vi "SaveConfigFile.vi"(0 "IP":string caption="Robot IP Address", 1 "RoboguideRobotPath":path, 2 "ConnectRoboguide":bool, 3 "Use Telnet":bool, 4 "Telnet password":string, 5 "Use FTP":bool, 6 "FTP user":string, 7 "FTP password":string, 8 "Use SNPX":bool, 9 "error in (no error)":errorcluster, 10 "Licensee":string, 12 "Key":string) -> ()   [LabVIEW 2019]
uses:
  <vilib>/Utility/config.llb/NI_LVConfig.lvlib
  <vilib>/Utility/config.llb/Write Key (Path).vi
  <vilib>/Utility/config.llb/Write Key (String).vi
  <vilib>/Utility/config.llb/Write Key (Boolean).vi
panel:
  out "error out":errorcluster
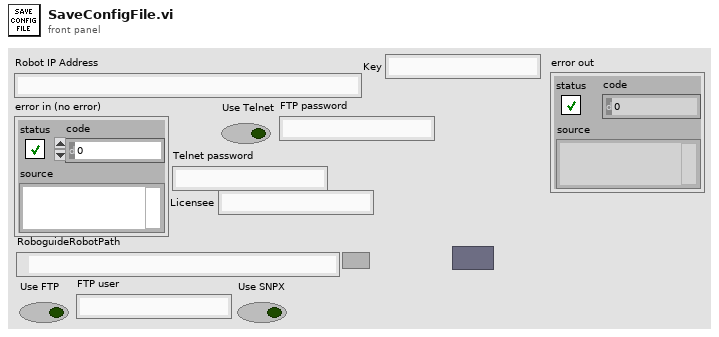
[diagram p1: front panel]
types:
  T1 = typedef "NI_LVConfig.lvlib/Config Data RefNum.ctl" = refnum<k1>
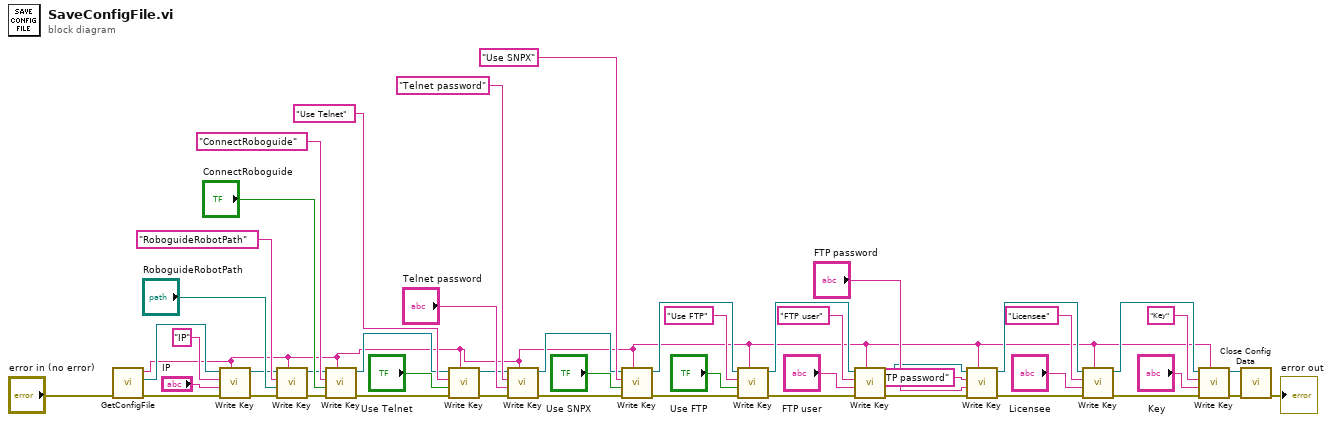
[diagram p0: block diagram]
diagram:
  n1 = call "GetConfigFile.vi"("error in (no error)"="error in (no error)") -> ("error out"=w48:errorcluster, "refnum"=w47:T1, "section"=w3:string)  [unwired: 8 in]
  n2 = call-poly <vilib>:"Write Key.vi"("section"=w3, "error in (no error)"=w48, "value"="IP", "key"="IP", "refnum"=w47) -> ("error out"=w15:errorcluster, "refnum out"=w1:T1)  [unwired: 4 in, 1 out]
  n3 = call-poly <vilib>:"Write Key.vi"("section"=w3, "error in (no error)"=w15, "value"="RoboguideRobotPath", "key"="RoboguideRobotPath", "refnum"=w1) -> ("error out"=w14:errorcluster, "refnum out"=w2:T1)  [unwired: 4 in, 1 out]
  n4 = call-poly <vilib>:"Write Key.vi"("section"=w3, "error in (no error)"=w14, "value"="ConnectRoboguide", "key"="ConnectRoboguide", "refnum"=w2) -> ("error out"=w13:errorcluster, "refnum out"=w16:T1)  [unwired: 4 in, 1 out]
  n5 = call-poly <vilib>:"Write Key.vi"("section"=w3, "error in (no error)"=w13, "value"="Use Telnet", "key"="Use Telnet", "refnum"=w16) -> ("error out"=w12:errorcluster, "refnum out"=w17:T1)  [unwired: 4 in, 1 out]
  n6 = call-poly <vilib>:"Write Key.vi"("section"=w3, "error in (no error)"=w12, "value"="Telnet password", "key"="Telnet password", "refnum"=w17) -> ("error out"=w11:errorcluster, "refnum out"=w18:T1)  [unwired: 4 in, 1 out]
  n7 = call-poly <vilib>:"Write Key.vi"("section"=w3, "error in (no error)"=w11, "value"="Use SNPX", "key"="Use SNPX", "refnum"=w18) -> ("error out"=w10:errorcluster, "refnum out"=w19:T1)  [unwired: 4 in, 1 out]
  n8 = call-poly <vilib>:"Write Key.vi"("section"=w3, "error in (no error)"=w10, "value"="Use FTP", "key"="Use FTP", "refnum"=w19) -> ("error out"=w9:errorcluster, "refnum out"=w20:T1)  [unwired: 4 in, 1 out]
  n9 = call-poly <vilib>:"Write Key.vi"("section"=w3, "error in (no error)"=w9, "value"="FTP user", "key"="FTP user", "refnum"=w20) -> ("error out"=w8:errorcluster, "refnum out"=w21:T1)  [unwired: 4 in, 1 out]
  n10 = call-poly <vilib>:"Write Key.vi"("section"=w3, "error in (no error)"=w8, "value"="FTP password", "key"="FTP password", "refnum"=w21) -> ("error out"=w7:errorcluster, "refnum out"=w22:T1)  [unwired: 4 in, 1 out]
  n11 = call-poly <vilib>:"Write Key.vi"("section"=w3, "error in (no error)"=w7, "value"="Licensee", "key"="Licensee", "refnum"=w22) -> ("error out"=w6:errorcluster, "refnum out"=w23:T1)  [unwired: 4 in, 1 out]
  n12 = call-poly <vilib>:"Write Key.vi"("section"=w3, "error in (no error)"=w6, "value"="Key", "key"="Key", "refnum"=w23) -> ("error out"=w5:errorcluster, "refnum out"=w24:T1)  [unwired: 4 in, 1 out]
  n13 = call <vilib>:"Close Config Data.vi"("error in (no error)"=w5, "refnum"=w24) -> ("error out"=→"error out":errorcluster)  [unwired: 8 in, 1 out]
